vi "Write Enable.vi"(7 "PWM":refnum<class "PWM.lvclass">, 8 "error in (no error)":errorcluster, 10 "Enable":bool, 11 "Session In":refnum<class "Session.lvclass">) -> (0 "error out":errorcluster, 3 "Session Out":refnum<class "Session.lvclass">)   [LabVIEW 2024, in "CTI.lvlib" / "PWM.lvclass"]
uses:
  PWM.lvclass
  Session/Session.lvclass
  PWM.lvclass/PWM.ctl
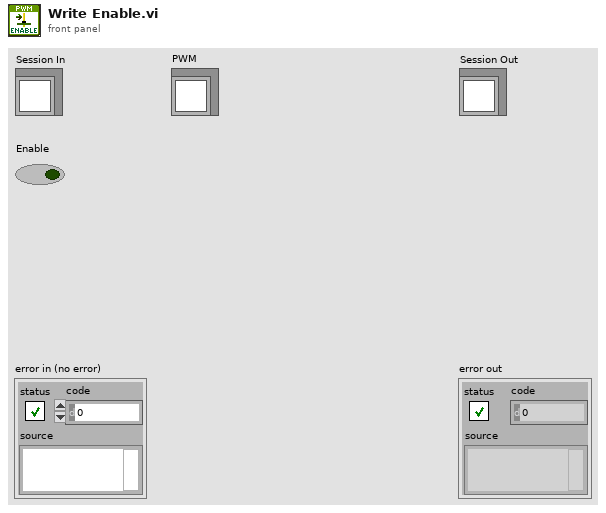
[diagram p1: front panel]
types:
  T1 = typedef "CTI.lvlib/GPIO Number.ctl" = i8
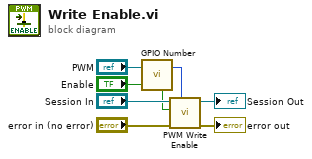
[diagram p0: block diagram]
diagram:
  n1 = call "GPIO Number.vi"("PWM in"="PWM") -> ("GPIO #"=w3:T1)  [unwired: 6 in]
  n2 = call "PWM Write Enable.vi"("GPIO #"=w3, "error in (no error)"="error in (no error)", "Enable"="Enable", "Session in"="Session In") -> ("error out"=→"error out":errorcluster, "Session out"=→"Session Out":refnum<class "Session.lvclass">)  [unwired: 6 in]
